vi "ZMQ Rep Test.vi"() -> ()   [LabVIEW 2019, in "RemoteControl.ZMQ.lvlib" / "RemoteControl.ZMQ.lvclass"]
uses:
  RemoteControl.ZMQ.lvclass
  C:/Program Files (x86)/National Instruments/LabVIEW 2019/user.lib/LevyLab/RemoteControl/RemoteControl/RemoteControl.lvclass
  <userlib>/LevyLab/RemoteControl/RemoteControl/RemoteControl.lvclass/RemoteControl.ctl
  <vilib>/addons/zeromq/zmq_context.lvclass
  <vilib>/addons/zeromq/socket_type.ctl
  <vilib>/addons/zeromq/zeromq.lvlib
  <vilib>/addons/zeromq/zmq_socket.lvclass
  <vilib>/addons/zeromq/socket_options.ctl
  <userlib>/LevyLab/RemoteControl/RemoteControl/RemoteControl.lvclass
panel:
  in  "stop":bool
  out "Command":string
  out "ID":string
  out "Data":variant
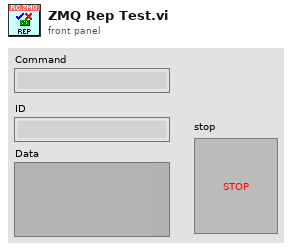
[diagram p1: front panel]
types:
  T1 = typedef "zeromq.lvlib/socket_options.ctl" = enum8{"NONE", "ZMQ_HWM", "<2>", "ZMQ_SWAP", "ZMQ_AFFINITY", "ZMQ_ROUTING_ID", "ZMQ_SUBSCRIBE", "ZMQ_UNSUBSCRIBE", "ZMQ_RATE", "ZMQ_RECOVERY_IVL", "ZMQ_MCAST_LOOP", "ZMQ_SNDBUF", "ZMQ_RCVBUF", "ZMQ_RCVMORE", "ZMQ_FD", "ZMQ_EVENTS", "ZMQ_TYPE", "ZMQ_LINGER", "ZMQ_RECONNECT_IVL", "ZMQ_BACKLOG", "ZMQ_RECOVERY_IVL_MSEC", "ZMQ_RECONNECT_IVL_MAX", "ZMQ_MAXMSGSIZE", "ZMQ_SNDHWM", "ZMQ_RCVHWM", "ZMQ_MULTICAST_HOPS", "<26>", "ZMQ_RCVTIMEO", "ZMQ_SNDTIMEO", "<29>", "<30>", "ZMQ_IPV4ONLY", "ZMQ_LAST_ENDPOINT", "ZMQ_ROUTER_MANDATORY", "ZMQ_TCP_KEEPALIVE", "ZMQ_TCP_KEEPALIVE_CNT", "ZMQ_TCP_KEEPALIVE_IDLE", "ZMQ_TCP_KEEPALIVE_INTVL", "ZMQ_TCP_ACCEPT_FILTER", "ZMQ_IMMEDIATE", "ZMQ_XPUB_VERBOSE", "ZMQ_ROUTER_RAW", "ZMQ_IPV6", "ZMQ_MECHANISM", "ZMQ_PLAIN_SERVER", "ZMQ_PLAIN_USERNAME", "ZMQ_PLAIN_PASSWORD", "ZMQ_CURVE_SERVER", "ZMQ_CURVE_PUBLICKEY", "ZMQ_CURVE_SECRETKEY", "ZMQ_CURVE_SERVERKEY", "ZMQ_PROBE_ROUTER", "ZMQ_REQ_CORRELATE", "ZMQ_REQ_RELAXED", "ZMQ_CONFLATE", "ZMQ_ZAP_DOMAIN", "ZMQ_ROUTER_HANDOVER", "ZMQ_TOS", "ZMQ_IPC_FILTER_PID", "ZMQ_IPC_FILTER_UID", "ZMQ_IPC_FILTER_GID", "ZMQ_CONNECT_ROUTING_ID", "ZMQ_GSSAPI_SERVER", "ZMQ_GSSAPI_PRINCIPAL", "ZMQ_GSSAPI_SERVICE_PRINCIPAL", "ZMQ_GSSAPI_PLAINTEXT", "ZMQ_HANDSHAKE_IVL", "<67>", "ZMQ_SOCKS_PROXY", "ZMQ_XPUB_NODROP", "ZMQ_BLOCKY", "ZMQ_XPUB_MANUAL", "ZMQ_XPUB_WELCOME_MSG", "ZMQ_STREAM_NOTIFY", "ZMQ_INVERT_MATCHING", "ZMQ_HEARTBEAT_IVL", "ZMQ_HEARTBEAT_TTL", "ZMQ_HEARTBEAT_TIMEOUT", "ZMQ_XPUB_VERBOSER", "ZMQ_CONNECT_TIMEOUT", "ZMQ_TCP_MAXRT", "ZMQ_THREAD_SAFE", "<82>", "<83>", "ZMQ_MULTICAST_MAXTPDU", "ZMQ_VMCI_BUFFER_SIZE", "ZMQ_VMCI_BUFFER_MIN_SIZE", "ZMQ_VMCI_BUFFER_MAX_SIZE", "ZMQ_VMCI_CONNECT_TIMEOUT", "ZMQ_USE_FD", "ZMQ_GSSAPI_PRINCIPAL_NAMETYPE", "ZMQ_GSSAPI_SERVICE_PRINCIPAL_NAMETYPE", "ZMQ_BINDTODEVICE", "ZMQ_ZAP_ENFORCE_DOMAIN", "ZMQ_LOOPBACK_FASTPATH", "ZMQ_METADATA", "ZMQ_MULTICAST_LOOP", "ZMQ_ROUTER_NOTIFY"}
  T2 = typedef "zeromq.lvlib/socket_type.ctl" = enum8{"ZMQ_PAIR", "ZMQ_PUB", "ZMQ_SUB", "ZMQ_REQ", "ZMQ_REP", "ZMQ_DEALER", "ZMQ_ROUTER", "ZMQ_PULL", "ZMQ_PUSH", "ZMQ_XPUB", "ZMQ_XSUB", "ZMQ_STREAM", "ZMQ_SERVER", "ZMQ_CLIENT", "ZMQ_RADIO", "ZMQ_DISH", "ZMQ_GATHER", "ZMQ_SCATTER", "ZMQ_DGRAM"}
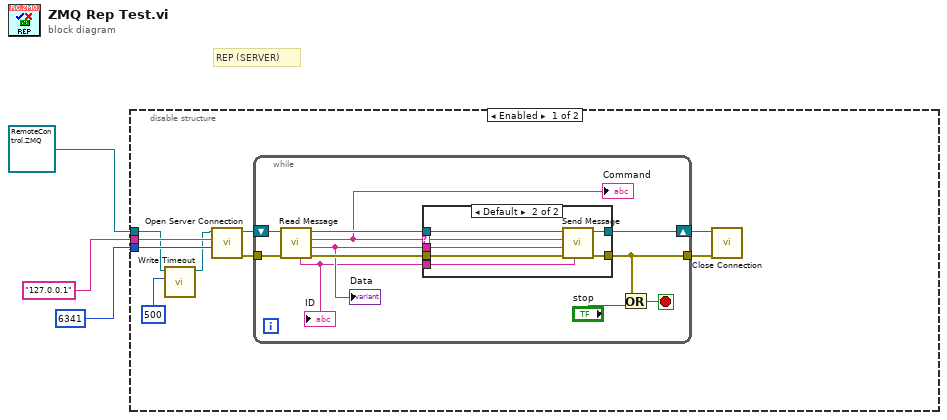
[diagram p0: block diagram]
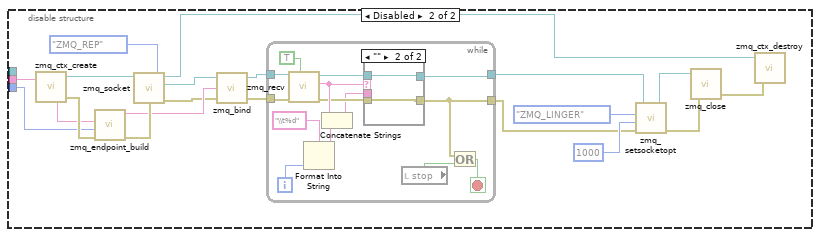
[diagram p3: hidden frame]
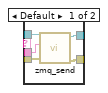
[diagram p4: hidden frame]
diagram:
  # "REP (SERVER)"
  n1 = disable-structure shown="Enabled" {
    disable-tunnel: refnum<class "RemoteControl.ZMQ.lvclass"> refnum ("RemoteControl.ZMQ.lvlib:RemoteControl.ZMQ.lvclass") -> [w5 _]
    disable-tunnel: u16 6341 ("Port") -> [w8 w40]
    disable-tunnel: "127.0.0.1" ("Address") -> [w7 w39]
    frame Enabled {
      n2 = call <userlib>:"Write Timeout.vi"("timeout (ms) [500]"=500 ("timeout in ms (100)"), "RemoteControl in"=w5) -> ("RemoteControl out"=w4:refnum<class "RemoteControl.ZMQ.lvclass">)  [unwired: 8 in, 1 out]
      n3 = call-dynamic "Open Server Connection.vi"("Port"=w8, "address"=w7, "RemoteControl.ZMQ in"=w4) -> ("error out"=w11:errorcluster, "RemoteControl.ZMQ out"=w12:refnum<class "RemoteControl.ZMQ.lvclass">)  [unwired: 7 in]
      n4 = while {
        tunnel: w11 -> [w22]
        tunnel: [w18] -> w9
        shift-right: [w19] -> w10
        shift-left: w12 -> [w23]
        stop <- w17 stop-if-true
        n5 = call-dynamic "Read Message.vi"("error in (no error)"=w22, "RemoteControl.ZMQ in"=w23) -> ("error out"=w21:errorcluster, "Data"=w14:string, "Command"=w15:string, "RemoteControl.ZMQ out"=w20:refnum<class "RemoteControl.ZMQ.lvclass">, "ID"=w13:string)  [unwired: 5 in]
        "Data" <- w14
        "ID" <- w13
        "Command" <- w15
        n6 = case shown="Default" w15 {
          selector: w15 -> [_ w27]
          tunnel: w21 -> [w24 w32]
          tunnel: w20 -> [w25 w31]
          tunnel: [w25 w30] -> w19
          tunnel: [w24 w29] -> w18
          tunnel: w13 -> [_ w28]
          tunnel: w14 -> [_ w26]
          frame "" {
            # "no incoming msg:\ndo nothing"
          }
          frame Default {
            n7 = call-dynamic "Send Message.vi"("ID"=w28, "error in (no error)"=w32, "Data"=w26, "Command"=w27, "RemoteControl.ZMQ in"=w31) -> ("error out"=w29:errorcluster, "RemoteControl.ZMQ out"=w30:refnum<class "RemoteControl.ZMQ.lvclass">)  [unwired: 5 in]
          }
        }
        n8 = Or(x=w18, y="stop") -> (x .or. y?=w17:bool)
      }
      n9 = call-dynamic "Close Connection.vi"("error in (no error)"=w9, "RemoteControl.ZMQ in"=w10) -> ()  [unwired: 8 in, 2 out]
    }
    frame Disabled {
      n10 = call <vilib>:"zmq_ctx_create.vi"() -> ("error out"=w49:errorcluster, "context out"=w51:refnum<class "zmq_context.lvclass">)  [unwired: 4 in]
      n11 = call <vilib>:"zmq_endpoint_build.vi"("error in"=w49, "port"=w40, "address"=w39) -> ("error out"=w48:errorcluster, "endpoint"=w37:string)  [unwired: 2 in, 1 out]
      n12 = call <vilib>:"zmq_socket.vi"("error in"=w48, "socket type"=socket_type."ZMQ_REP", "context in"=w51) -> ("error out"=w36:errorcluster, "socket out"=w38:refnum<class "zmq_socket.lvclass">, "context out"=w41:refnum<class "zmq_context.lvclass">)  [unwired: 2 in]
      n13 = call <vilib>:"zmq_bind.vi"("error in"=w36, "endpoint"=w37, "socket in"=w38) -> ("error out"=w34:errorcluster, "socket out"=w35:refnum<class "zmq_socket.lvclass">)  [unwired: 1 in]
      n14 = while {
        tunnel: w34 -> [w62]
        tunnel: w35 -> [w63]
        tunnel: [w60] -> w44
        tunnel: [w55] -> w33
        i -> [w58]
        stop <- w64 stop-if-true
        n15 = call <vilib>:"zmq_recv.vi"("no block? (F)"=TRUE, "error in"=w62, "socket in"=w63) -> ("error out"=w53:errorcluster, "data"=w54:string, "socket out"=w61:refnum<class "zmq_socket.lvclass">)  [unwired: 2 in, 2 out]
        n16 = Format Into String(format string="\\t%d" ("Command"), w58) -> (resulting string=w57:string)  [unwired: 2 in, 1 out]
        n17 = Concatenate Strings(w54, w57) -> (w52:string)
        n18 = case shown="\"\"" w54 {
          tunnel: w61 -> [w70 w72]
          tunnel: [w69 w72] -> w60
          tunnel: [w68 w71] -> w55
          tunnel: w53 -> [w66 w71]
          tunnel: w52 -> [w67 _]
          frame Default {
            n19 = call <vilib>:"zmq_send.vi"("error in"=w66, "data"=w67, "socket in"=w70) -> ("error out"=w68:errorcluster, "socket out"=w69:refnum<class "zmq_socket.lvclass">)  [unwired: 4 in]
          }
          frame "" {
          }
        }
        n20 = local read "stop"() -> (w65:bool)
        n21 = Or(x=w55, y=w65) -> (x .or. y?=w64:bool)
      }
      n22 = call <vilib>:"zmq_setsocketopt.vi"("error in"=w33, "value"=1000, "option"=socket_options."ZMQ_LINGER", "socket in"=w44) -> ("error out"=w43:errorcluster, "socket out"=w45:refnum<class "zmq_socket.lvclass">)  [unwired: 2 in]
      n23 = call <vilib>:"zmq_close.vi"("error in"=w43, "socket"=w45) -> ("error out"=w42:errorcluster)  [unwired: 3 in]
      n24 = call <vilib>:"zmq_ctx_destroy.vi"("error in"=w42, "context in"=w41) -> ()  [unwired: 3 in, 1 out]
    }
  }
